vi "MNK_FP_to_DSC.vi"(0 "str":string[](array[string]), 1 "str var":refnum<k21>[](array[refnum])=["ni.var.psp://housesoftheholy/MNK_18T/MNK_FP_STATE"], 2 "dbl":dbl[](array[numeric]), 3 "dbl var":refnum<k21>[](array[refnum])=["ni.var.psp://housesoftheholy/MNK_18T/MNK_FP_P1", "ni.var.psp://housesoftheholy/MNK_18T/MNK_FP_P2", "ni.var.psp://housesoftheholy/MNK_18T/MNK_FP_P3", "ni.var.psp://housesoftheholy/MNK_18T/MNK_FP_P4", "ni.var.psp://housesoftheholy/MNK_18T/MNK_FP_P5", "ni.var.psp://housesoftheholy/MNK_18T/MNK_FP_P6", "ni.var.psp://housesoftheholy/MNK_18T/MNK_FP_P7", "ni.var.psp://housesoftheholy/MNK_18T/MNK_FP_Flow", "ni.var.psp://housesoftheholy/MNK_18T/MNK_FP_MG0", "ni.var.psp://housesoftheholy/MNK_18T/MNK_FP_MG1", "ni.var.psp://housesoftheholy/MNK_18T/MNK_FP_MG2", "ni.var.psp://housesoftheholy/MNK_18T/MNK_FP_MG3", "ni.var.psp://housesoftheholy/MNK_18T/MNK_FP_MG4", "ni.var.psp://housesoftheholy/MNK_18T/MNK_FP_MG5", "ni.var.psp://housesoftheholy/MNK_18T/MNK_FP_state0", "ni.var.psp://housesoftheholy/MNK_18T/MNK_FP_state1", "ni.var.psp://housesoftheholy/MNK_18T/MNK_FP_state2"]) -> ()   [LabVIEW 2016]
panel:
  out "error out":errorcluster
  in  "error in (no error)":errorcluster
  # "MNK FP to DSC"
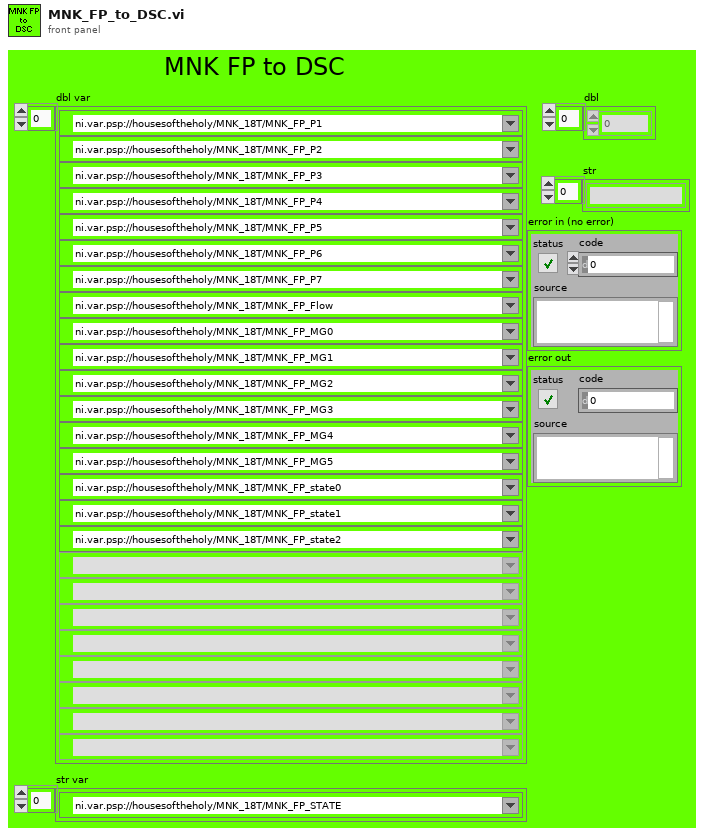
[diagram p1: front panel]
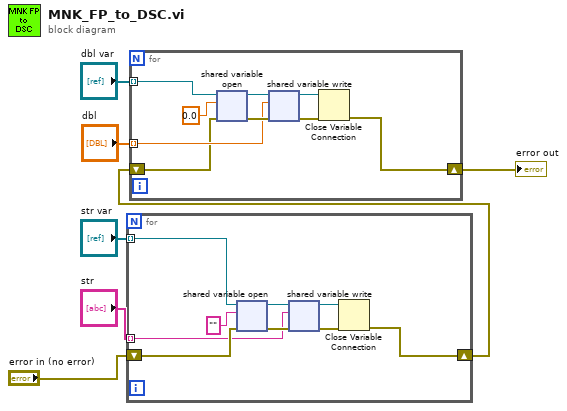
[diagram p0: block diagram]
diagram:
  n1 = for {
    tunnel: "str var" -> [w10] mode=indexing
    tunnel: "str" -> [w9] mode=indexing
    shift-right: [w8] -> w1
    shift-left: "error in (no error)" -> [w11]
    n2 = shared-variable-open(w10, w11, "") -> (w14:refnum<k21>, w15:errorcluster)  [unwired: 1 in]
    n3 = shared-variable-write(w14, w15, w9) -> (w13:refnum<k21>, w16:errorcluster)
    n4 = Close Variable Connection(8:w16, 11:w13) -> (0:w8:errorcluster)
  }
  n5 = for {
    tunnel: "dbl var" -> [w18] mode=indexing
    tunnel: "dbl" -> [w20] mode=indexing
    shift-right: [w17] -> w2
    shift-left: w1 -> [w19]
    n6 = shared-variable-open(w18, w19, 0.0) -> (w23:refnum<k21>, w24:errorcluster)  [unwired: 1 in]
    n7 = shared-variable-write(w23, w24, w20) -> (w22:refnum<k21>, w25:errorcluster)
    n8 = Close Variable Connection(8:w25, 11:w22) -> (0:w17:errorcluster)
  }
  "error out" <- w2
